vi "Run SV process.vi"(8 "error in (no error)":errorcluster, 11 "SV Data":T1={"Status notifier"=refnum, "Write FIFO ref"=refnum, "Read FIFO ref"=refnum, "Status FIFO ref"=refnum, "Update Rate"=1, "Write Refs by Type"={"DBL Write"=[]}, "Read Refs by Type"={"DBL Read"=[]}, "WriteSize"=0, "ReadSize"=0}) -> (0 "error out":errorcluster, 3 "SV Data":T1={"Status notifier"=refnum, "Write FIFO ref"=refnum, "Read FIFO ref"=refnum, "Status FIFO ref"=refnum, "Update Rate"=1, "Write Refs by Type"={"DBL Write"=[]}, "Read Refs by Type"={"DBL Read"=[]}, "WriteSize"=0, "ReadSize"=0})   [LabVIEW 2020, in "Shared Variable Interface.lvlib"]
uses:
  Shared Variable Interface.lvlib
  SV Process Configuration.ctl
  SVGlobal_StatusStop.vi
  SVGlobal_WriteStat.vi
  SVGlobal_ReadStat.vi
  DataTypes/DBL/WriteSV.vi
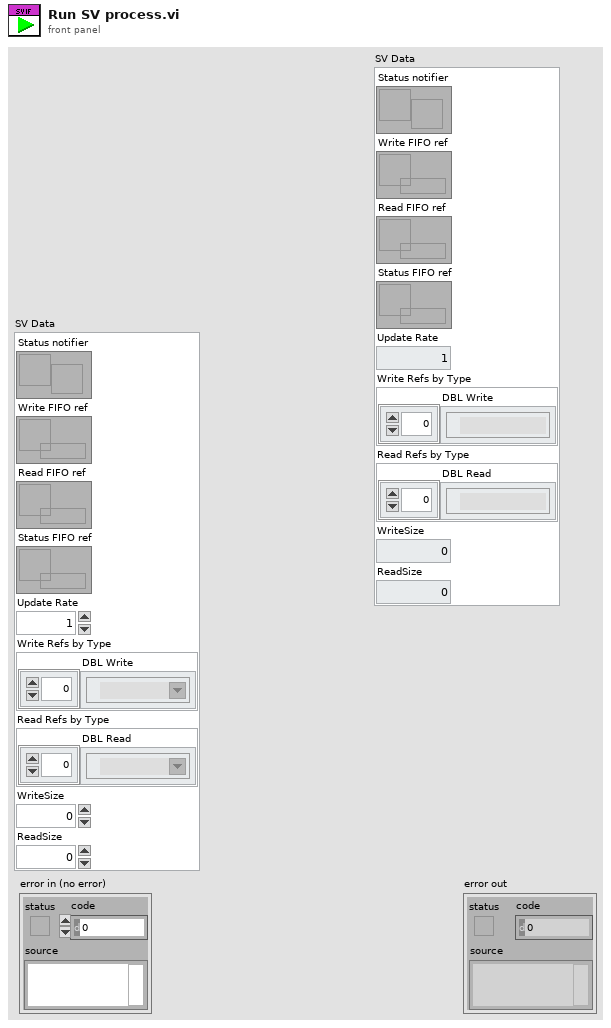
[diagram p1: front panel]
types:
  T1 = typedef "Shared Variable Interface.lvlib/SV Process Configuration.ctl" = cluster{"Status notifier":refnum<notifier>, "Write FIFO ref":refnum<k33>, "Read FIFO ref":refnum<k33>, "Status FIFO ref":refnum<k33>, "Update Rate":u32, "Write Refs by Type":cluster{"DBL Write":refnum<k21>[]}, "Read Refs by Type":cluster{"DBL Read":refnum<k21>[]}, "WriteSize":i32, "ReadSize":i32}
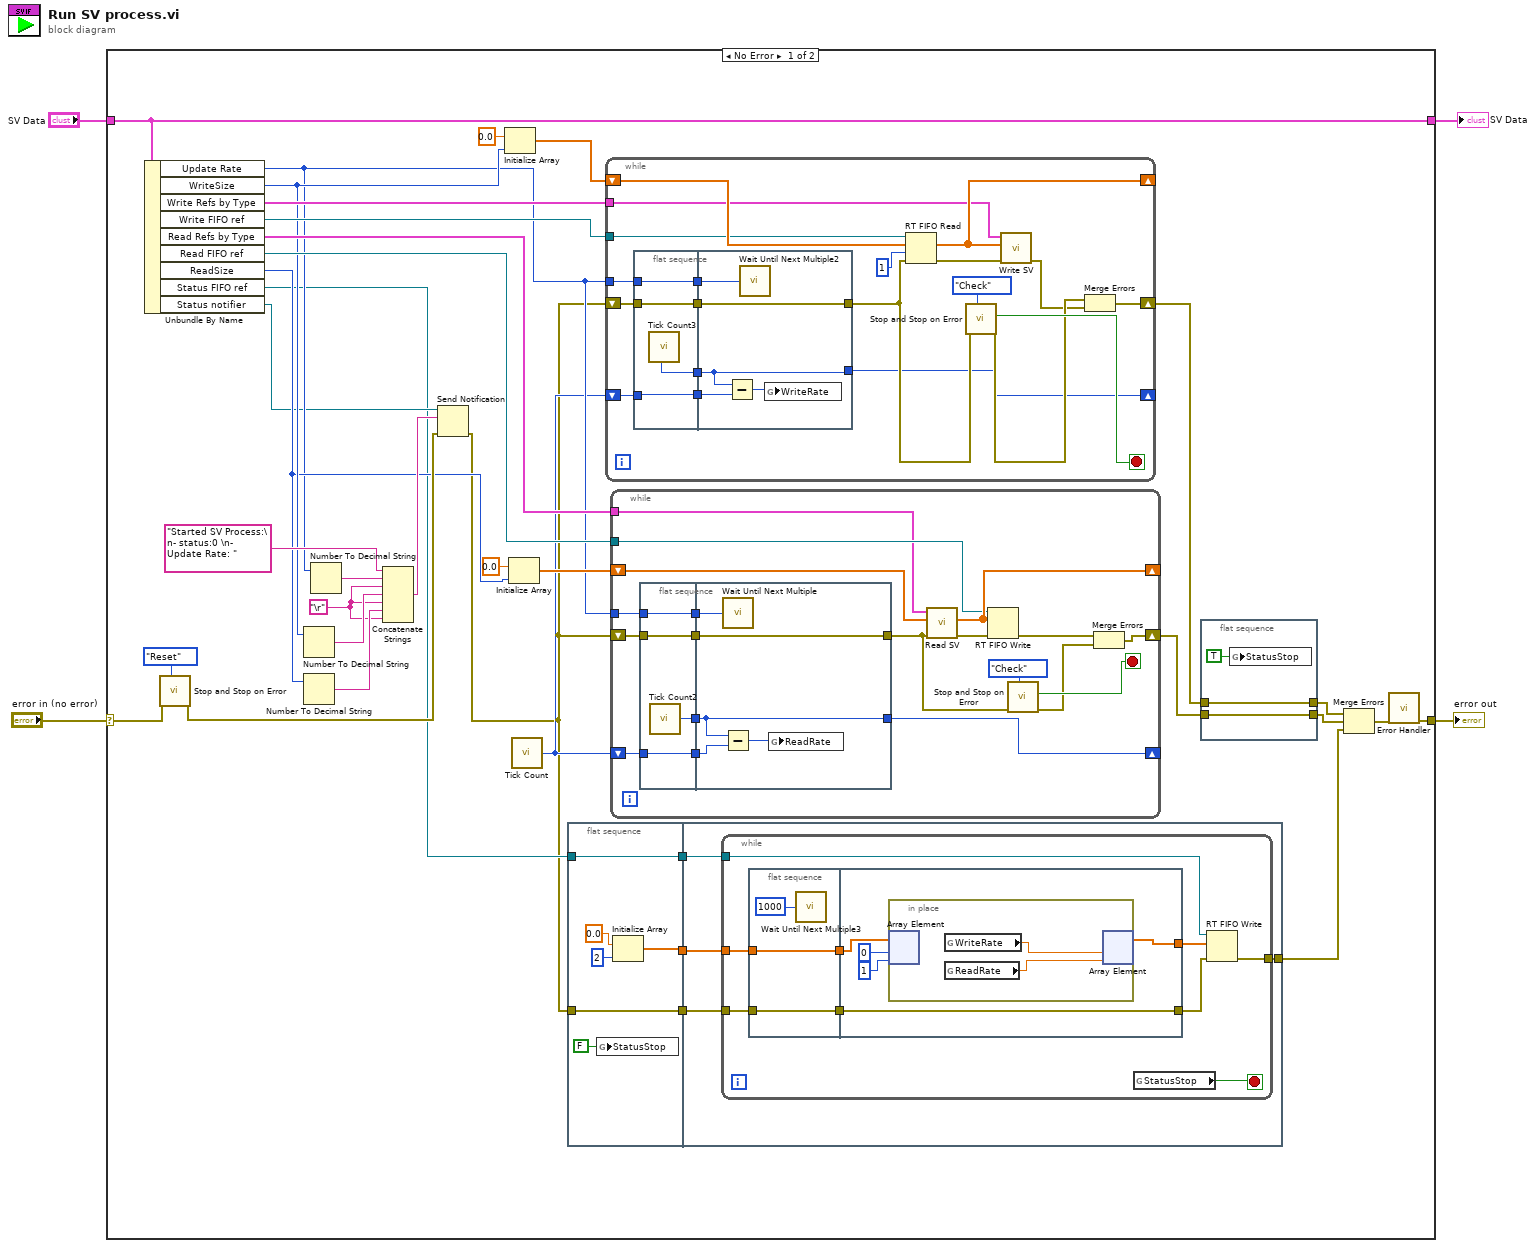
[diagram p0: block diagram]
diagram:
  n1 = case shown="No Error" "error in (no error)" {
    selector: "error in (no error)" -> [w34 w130]
    tunnel: [w35 w130] -> w3
    tunnel: "SV Data" -> [w21 w129]
    tunnel: [w21 w129] -> w1
    frame No Error {
      w23 = "\r" ("string")
      n2 = Unbundle By Name(w21) -> ("Update Rate"=w18:u32, "WriteSize"=w20:i32, "Write Refs by Type"=w29:cluster{"DBL Write":refnum<k21>[]}, "Write FIFO ref"=w39:refnum<k33>, "Read Refs by Type"=w30:cluster{"DBL Read":refnum<k21>[]}, "Read FIFO ref"=w31:refnum<k33>, "ReadSize"=w19:i32, "Status FIFO ref"=w14:refnum<k33>, "Status notifier"=w15:refnum<notifier>)
      n3 = call "Stop and Stop on Error.vi"("Action"=enum16{"Check", "Reset"}."Reset", "error in (no error)"=w34) -> ("error out"=w22:errorcluster)  [unwired: 8 in, 1 out]
      n4 = Number To Decimal String(number=w20) -> (decimal integer string=w25:string)  [unwired: 1 in]
      n5 = Number To Decimal String(number=w19) -> (decimal integer string=w24:string)  [unwired: 1 in]
      n6 = Number To Decimal String(number=w18) -> (decimal integer string=w32:string)  [unwired: 1 in]
      n7 = Concatenate Strings("Started SV Process:\n- status:0 \n- Update Rate: " ("notification"), w32, w23, w25, w23, w24, w23) -> (w33:string)
      n8 = Send Notification(notification=w33, notifier=w15, error in (no error)=w22) -> (error out=w13:errorcluster)  [unwired: 1 out]
      n9 = Initialize Array(0.0 ("element"), w20) -> (w27:dbl[])
      n10 = Initialize Array(0.0 ("element"), w19) -> (w26:dbl[])
      n11 = call "Tick Count"() -> ("Tick Count(uSec)"=w16:u32)
      n12 = flat-sequence {
        tunnel: w13 -> [w44]
        tunnel: w14 -> [w45]
        tunnel: [w45] -> w7
        tunnel: [w44] -> w6
        tunnel: [w41] -> w5
        tunnel: [w46] -> w12
        tunnel: w7 -> [w49]
        tunnel: w6 -> [w48]
        tunnel: w5 -> [w47]
        frame #0 {
          n13 = global write "SVGlobal_StatusStop.vi" "StatusStop"(FALSE) -> ()
          n14 = Initialize Array(0.0, 2 ("dimension size")) -> (w41:dbl[])
        }
        frame #1 {
          n15 = while {
            tunnel: w49 -> [w58]
            tunnel: w48 -> [w57]
            tunnel: w47 -> [w53]
            tunnel: [w52] -> w46
            stop <- w50 stop-if-true
            n16 = flat-sequence {
              tunnel: w57 -> [w60]
              tunnel: [w60] -> w56
              tunnel: [w59] -> w54
              tunnel: w53 -> [w59]
              tunnel: [w66] -> w55
              tunnel: w56 -> [w66]
              tunnel: w54 -> [w65]
              tunnel: [w64] -> w51
              frame #0 {
                n17 = call "Wait Until Next Multiple3"("Count(mSec)"=u32 1000 ("Count(uSec)")) -> ()  [unwired: 1 out]
              }
              frame #1 {
                n18 = in-place {
                  n19 = in-place-array #1(w65, 0, 1) -> ()  [unwired: 2 out]
                  n20 = global read "SVGlobal_WriteStat.vi" "WriteRate"() -> (w68:dbl)
                  n21 = global read "SVGlobal_ReadStat.vi" "ReadRate"() -> (w67:dbl)
                  n22 = in-place-array #1(w68, w67) -> (w64:dbl[])  [unwired: 2 out]
                }
              }
            }
            n23 = global read "SVGlobal_StatusStop.vi" "StatusStop"() -> (w50:bool)
            n24 = RT FIFO Write(0:w58, 1:w51, 3:w55) -> (11:w52:errorcluster)  [unwired: 2 in, 3 out]
          }
        }
      }
      n25 = while {
        tunnel: w39 -> [w78]
        shift-right: [w81] -> w10
        shift-left: w13 -> [w89]
        tunnel: w18 -> [w88]
        tunnel: w29 -> [w79]
        shift-right: [w85] -> _
        shift-left: w27 -> [w86]
        shift-right: [w73] -> _
        shift-left: w16 -> [w75]
        stop <- w91 stop-if-true
        n26 = flat-sequence {
          tunnel: w88 -> [w94]
          tunnel: w89 -> [w95]
          tunnel: [w95] -> w77
          tunnel: [w94] -> w76
          tunnel: w75 -> [w92]
          tunnel: [w93] -> w74
          tunnel: [w92] -> w72
          tunnel: [w100] -> w80
          tunnel: w77 -> [w100]
          tunnel: w76 -> [w99]
          tunnel: w74 -> [w98]
          tunnel: [w98] -> w73
          tunnel: w72 -> [w97]
          frame #0 {
            n27 = call "Tick Count3"() -> ("Tick Count(uSec)"=w93:u32)
          }
          frame #1 {
            n28 = Subtract(x=w98, y=w97) -> (x-y=w96:u32)
            n29 = call "Wait Until Next Multiple2"("Count(uSec)"=w99) -> ()  [unwired: 1 out]
            n30 = global write "SVGlobal_WriteStat.vi" "WriteRate"(w96) -> ()
          }
        }
        n31 = RT FIFO Read(0:w78, 1:w86, 2:1 ("timeout in ms (0)"), 3:w80) -> (9:w85:dbl[], 11:w84:errorcluster)  [unwired: 3 out]
        n32 = call "Stop and Stop on Error.vi"("Action"=enum16{"Check", "Reset"}."Check", "error in (no error)"=w80) -> ("error out"=w83:errorcluster, "Stop?"=w91:bool)  [unwired: 8 in]
        n33 = call "Write SV.vi"("error in (no error)"=w84, "Data"=w85, "Write Refs by Type"=w79) -> ("error out"=w82:errorcluster)  [unwired: 8 in]
        n34 = Merge Errors(w83, w82) -> (w81:errorcluster)
      }
      n35 = while {
        tunnel: w31 -> [w112]
        shift-right: [w113] -> w8
        shift-left: w13 -> [w109]
        tunnel: w18 -> [w108]
        tunnel: w30 -> [w111]
        shift-right: [w116] -> _
        shift-left: w26 -> [w115]
        shift-right: [w102] -> _
        shift-left: w16 -> [w104]
        stop <- w118 stop-if-true
        n36 = flat-sequence {
          tunnel: w108 -> [w122]
          tunnel: w109 -> [w123]
          tunnel: [w123] -> w107
          tunnel: [w122] -> w106
          tunnel: [w121] -> w105
          tunnel: w104 -> [w120]
          tunnel: [w120] -> w103
          tunnel: [w128] -> w110
          tunnel: w107 -> [w128]
          tunnel: w106 -> [w127]
          tunnel: w105 -> [w125]
          tunnel: w103 -> [w126]
          tunnel: [w125] -> w102
          frame #0 {
            n37 = call "Tick Count2"() -> ("Tick Count(uSec)"=w121:u32)
          }
          frame #1 {
            n38 = call "Wait Until Next Multiple"("Count(uSec)"=w127) -> ()  [unwired: 1 out]
            n39 = Subtract(x=w125, y=w126) -> (x-y=w124:u32)
            n40 = global write "SVGlobal_ReadStat.vi" "ReadRate"(w124) -> ()
          }
        }
        n41 = call "Read SV.vi"("error in (no error)"=w110, "Data"=w115, "Read Refs by Type"=w111) -> ("error out"=w114:errorcluster, "Data Out"=w116:dbl[])  [unwired: 7 in]
        n42 = RT FIFO Write(0:w112, 1:w116, 3:w114) -> (11:w101:errorcluster)  [unwired: 2 in, 3 out]
        n43 = call "Stop and Stop on Error.vi"("Action"=enum16{"Check", "Reset"}."Check", "error in (no error)"=w110) -> ("error out"=w117:errorcluster, "Stop?"=w118:bool)  [unwired: 8 in]
        n44 = Merge Errors(w101, w117) -> (w113:errorcluster)
      }
      n45 = flat-sequence {
        tunnel: [w71] -> w11
        tunnel: w10 -> [w71]
        tunnel: [w70] -> w9
        tunnel: w8 -> [w70]
        frame #0 {
          n46 = global write "SVGlobal_StatusStop.vi" "StatusStop"(TRUE) -> ()
        }
      }
      n47 = Merge Errors(w11, w9, w12) -> (w36:errorcluster)
      n48 = call "Error Handler.vi"("error in (no error)"=w36) -> ("error out"=w35:errorcluster)  [unwired: 10 in]
    }
    frame Error {
    }
  }
  "error out" <- w3
  "SV Data" <- w1
